vi "AnalogTrigger.vi"(0 "UpperLimit":u32, 1 "LowerLimit":u32, 2 "DutyCycles":fxp<+/-,31,31>[](array[numeric])=[0.0, 0.0, 0.0, 0.0, 0.0, 0.0, 0.0, 0.0], 3 "AnalogInputs":u16[](array[numeric])=[0, 0, 0, 0, 0, 0, 0, 0], 4 "SourceSelect":T1) -> (5 "Output":T2)   [LabVIEW 2019]
uses:
  Helpers/AnalogTriggerOutput.ctl
  <vilib>/rvi/Emulation/niFpgaSctlEmulationGetInTimedLoop.vi
  <vilib>/rvi/Emulation/niFpgaProcessEmulError.vi
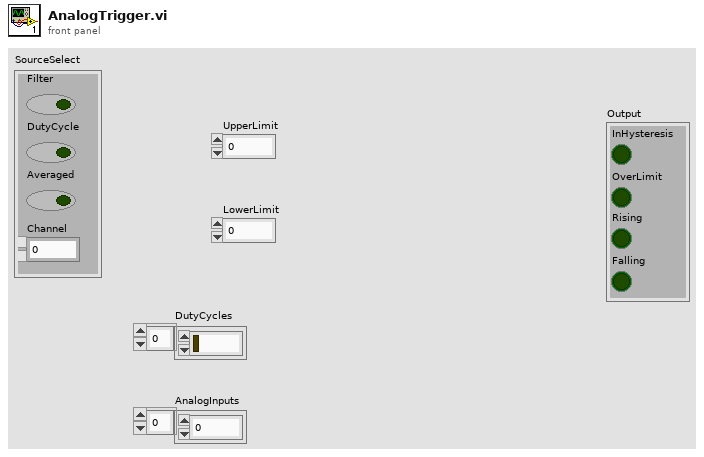
[diagram p1: front panel]
types:
  T1 = cluster{"Filter":bool, "DutyCycle":bool, "Averaged":bool, "Channel":fxp<+,3,3>}
  T2 = typedef "AnalogTriggerOutput.ctl" = cluster{"InHysteresis":bool, "OverLimit":bool, "Rising":bool, "Falling":bool}
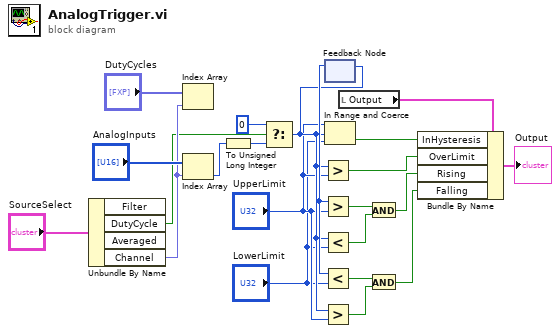
[diagram p0: block diagram]
diagram:
  n1 = Unbundle By Name("SourceSelect") -> ("DutyCycle"=w18:bool, "Channel"=w19:fxp<+,3,3>)  [unwired: 2 out]
  n2 = Index Array(array="DutyCycles", index=w19) -> ()  [unwired: 1 out]
  n3 = Index Array(array="AnalogInputs", index=w19) -> (element=w3:u16)
  n4 = To Unsigned Long Integer(number=w3) -> (unsigned 32bit integer=w2:u32)
  n5 = Select(t=u32 0, s=w18, f=w2) -> (s? t:f=w7:u32)
  n6 = Greater?(x=w7, y="UpperLimit") -> (0:w8:bool)
  n7 = Less?(x=w7, y="LowerLimit") -> (x < y?=w16:bool)
  n8 = Greater?(x=w7, y="UpperLimit") -> (0:w10:bool)
  n9 = feedback-in #1(w7) -> ()
  n10 = feedback #1() -> (w12:u32)  [unwired: 1 in]
  n11 = Greater?(x=w12, y="UpperLimit") -> (0:w17:bool)
  n12 = Less?(x=w12, y="LowerLimit") -> (x < y?=w11:bool)
  n13 = In Range and Coerce(upper limit="UpperLimit", x=w7, lower limit="LowerLimit") -> (In Range?=w4:bool)  [unwired: 1 out]
  n14 = local read "Output"() -> (w14:T2)
  n15 = And(x=w17, y=w16) -> (x .and. y?=w13:bool)
  n16 = And(x=w11, y=w10) -> (x .and. y?=w9:bool)
  n17 = Bundle By Name(cluster=w14, "InHysteresis"=w4, "OverLimit"=w8, "Rising"=w13, "Falling"=w9) -> (→"Output":T2)
